vi "Fetch Computer ID (SubVI).vi"(8 "Error in (no error)":errorcluster, 11 "VI Reference":refnum<vi>) -> (0 "Error out":errorcluster, 3 "Computer ID":string)   [LabVIEW 2022 SP3]
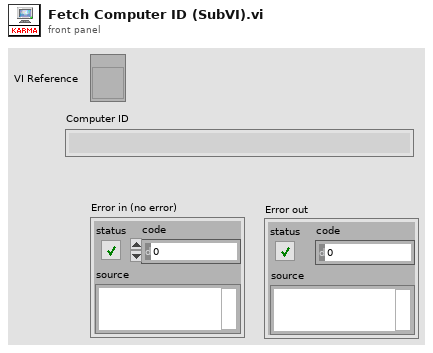
[diagram p1: front panel]
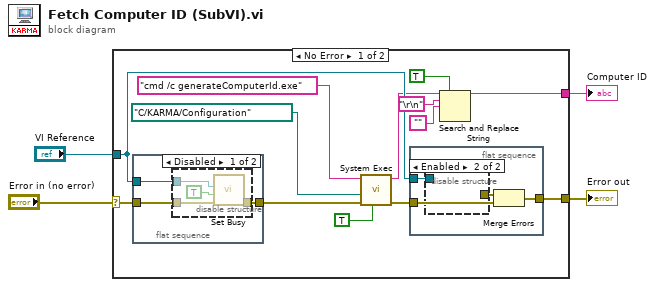
[diagram p0: block diagram]
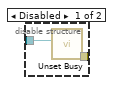
[diagram p2: hidden frame]
diagram:
  n1 = case shown="No Error" "Error in (no error)" {
    selector: "Error in (no error)" -> [w15 w31]
    tunnel: [w12 w31] -> w3
    tunnel: "VI Reference" -> [w11 _]
    tunnel: [w7 _] -> w1
    frame No Error {
      n2 = flat-sequence {
        tunnel: w15 -> [w26]
        tunnel: [w25] -> w14
        tunnel: w11 -> [w24]
        frame #0 {
          n3 = disable-structure shown="Disabled" {
            disable-tunnel: w26 -> [w30 _]
            disable-tunnel: [w29 _] -> w25
            disable-tunnel: w24 -> [w28 _]
            frame Disabled {
              n4 = call <vilib>:"Set Busy.vi"("error in (no error)"=w30, "disable click? (T)"=TRUE, "VI reference (current VI)"=w28) -> ("error out"=w29:errorcluster)  [unwired: 7 in, 1 out]
            }
            frame Enabled {
            }
          }
        }
      }
      n5 = call <vilib>:"System Exec.vi"("run minimized? (F)"=TRUE, "error in (no error)"=w14, "working directory"=path "C:/KARMA/Configuration", "command line"="cmd /c generateComputerId.exe") -> ("error out"=w13:errorcluster, "standard output"=w8:string)  [unwired: 4 in, 2 out]
      n6 = flat-sequence {
        tunnel: w13 -> [w21]
        tunnel: [w19] -> w12
        tunnel: w11 -> [w18]
        frame #0 {
          n7 = disable-structure shown="Enabled" {
            disable-tunnel: [w23 _] -> w20
            disable-tunnel: w18 -> [w22 _]
            frame Disabled {
              n8 = call <vilib>:"Unset Busy.vi"("VI reference (current VI)"=w22) -> ("error out"=w23:errorcluster)  [unwired: 10 in]
            }
            frame Enabled {
            }
          }
          n9 = Merge Errors(w20, w21) -> (w19:errorcluster)
        }
      }
      n10 = Search and Replace String(replace all?=TRUE ("replace all? (F)"), input string=w8, search string="\r\n", replace string="") -> (result string=w7:string)  [unwired: 4 in, 3 out]
    }
    frame Error {
    }
  }
  "Error out" <- w3
  "Computer ID" <- w1
